vi "Microtrabajo_3.vi"() -> ()   [LabVIEW 2022 SP3]
panel:
  in  "?":enum32{" 1", "2"}(tab)
  in  "?":bool
  out "Fibonacci":string
  in  "Valor límite":dbl
  in  "Stop Button":bool
  in  "DECREMENTAR":bool
  in  "INCREMENTAR":bool
  out "ITERACIONES":string
  out "CUENTA":string
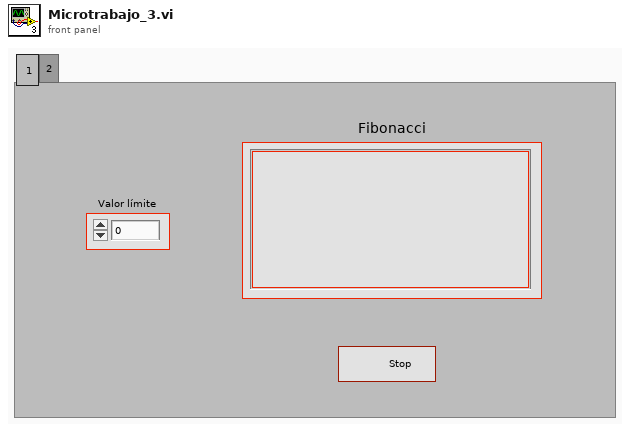
[diagram p1: front panel]
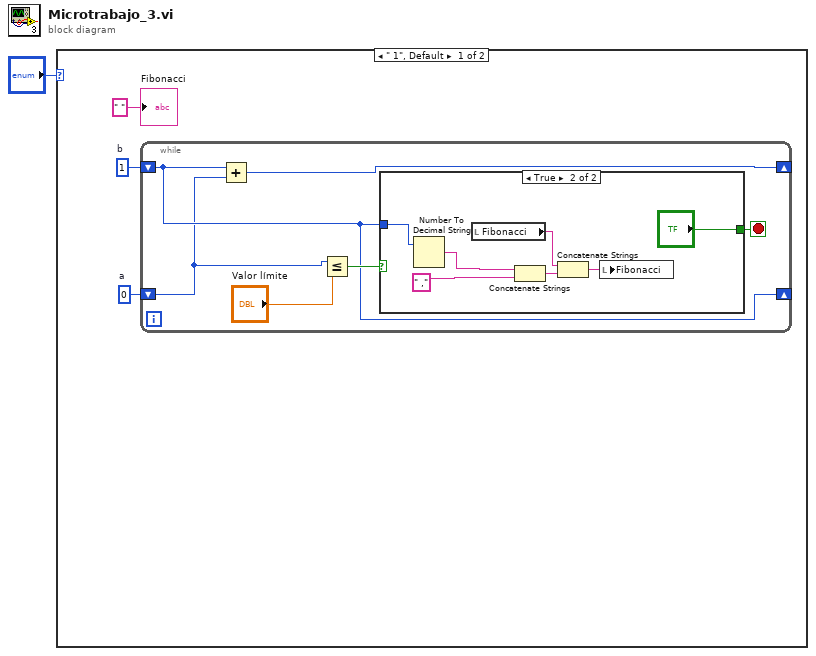
[diagram p0: block diagram]
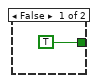
[diagram p2: hidden frame]
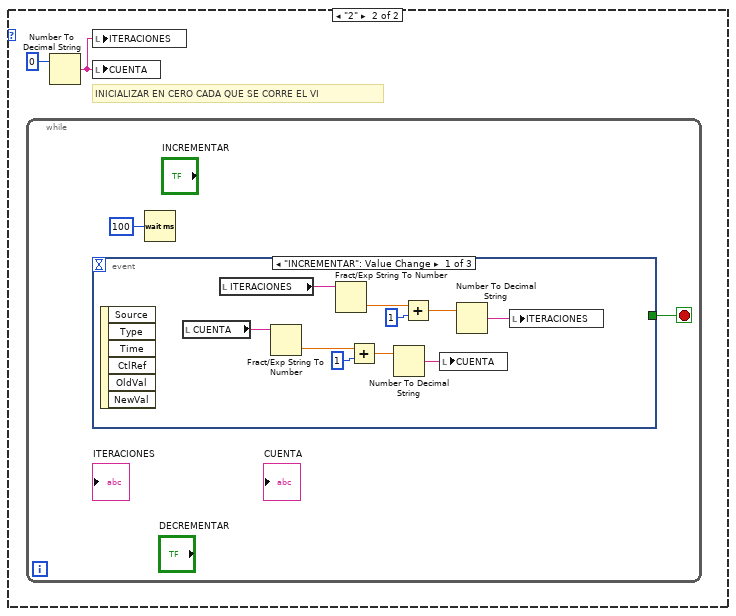
[diagram p3: hidden frame]
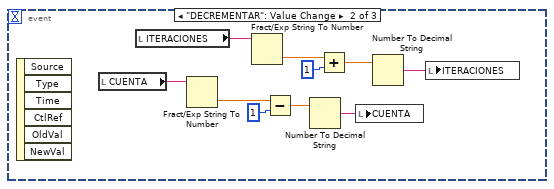
[diagram p4: hidden frame]
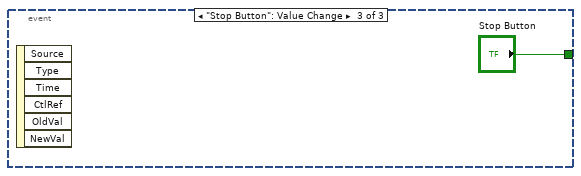
[diagram p5: hidden frame]
diagram:
  n1 = case shown="\" 1\", Default" "?" {
    frame " 1", Default {
      w3 = 0  # a
      w4 = 1  # b
      n2 = while {
        shift-right: [w8] -> _
        shift-left: w4 -> [w7]
        shift-right: [w7] -> _
        shift-left: w3 -> [w5]
        stop <- w6 stop-if-true
        n3 = Add(x=w7, y=w5) -> (x+y=w8:i32)
        n4 = Less Or Equal?(x=w5, y="Valor límite") -> (x <= y?=w9:bool)
        n5 = case shown="True" w9 {
          tunnel: w7 -> [_ w18]
          tunnel: [TRUE "?"] -> w6
          frame False {
          }
          frame True {
            n6 = Number To Decimal String(number=w18) -> (decimal integer string=w12:string)  [unwired: 1 in]
            n7 = local read "Fibonacci"() -> (w15:string)
            n8 = Concatenate Strings(w12, " ,") -> (w14:string)
            n9 = Concatenate Strings(w15, w14) -> (w16:string)
            n10 = local write "Fibonacci"(w16) -> ()
          }
        }
      }
      "Fibonacci" <- " "
    }
    frame "2" {
      # "INICIALIZAR EN CERO CADA QUE SE CORRE EL VI"
      n11 = while {
        stop <- w21 stop-if-true
        n12 = event shown="[0] \"INCREMENTAR\": Value Change" {
          selector: _ -> [_ _ _]
          dyn-events: _ -> [_ _ _]
          timeout: _ -> [_ _ _]
          tunnel: [_ _ "Stop Button"] -> w21
          event "INCREMENTAR": Value Change {
            n13 = event-data() -> ()  [unwired: 1 in, 6 out]
            n14 = local read "CUENTA"() -> (w28:string)
            n15 = local read "ITERACIONES"() -> (w30:string)
            n16 = Fract/Exp String To Number(string=w28) -> (number=w27:dbl)  [unwired: 3 in, 1 out]
            n17 = Fract/Exp String To Number(string=w30) -> (number=w29:dbl)  [unwired: 3 in, 1 out]
            n18 = Add(x=w27, y=1) -> (x+y=w26:dbl)
            n19 = Number To Decimal String(number=w26) -> (decimal integer string=w25:string)  [unwired: 1 in]
            n20 = Add(x=w29, y=1) -> (x+y=w24:dbl)
            n21 = local write "CUENTA"(w25) -> ()
            n22 = Number To Decimal String(number=w24) -> (decimal integer string=w23:string)  [unwired: 1 in]
            n23 = local write "ITERACIONES"(w23) -> ()
          }
          event "DECREMENTAR": Value Change {
            n24 = event-data() -> ()  [unwired: 1 in, 6 out]
            n25 = local read "CUENTA"() -> (w40:string)
            n26 = local read "ITERACIONES"() -> (w42:string)
            n27 = Fract/Exp String To Number(string=w40) -> (number=w35:dbl)  [unwired: 3 in, 1 out]
            n28 = Fract/Exp String To Number(string=w42) -> (number=w41:dbl)  [unwired: 3 in, 1 out]
            n29 = Subtract(x=w35, y=1) -> (x-y=w33:dbl)
            n30 = Number To Decimal String(number=w33) -> (decimal integer string=w39:string)  [unwired: 1 in]
            n31 = Add(x=w41, y=1) -> (x+y=w38:dbl)
            n32 = local write "CUENTA"(w39) -> ()
            n33 = Number To Decimal String(number=w38) -> (decimal integer string=w37:string)  [unwired: 1 in]
            n34 = local write "ITERACIONES"(w37) -> ()
          }
          event "Stop Button": Value Change {
            n35 = event-data() -> ()  [unwired: 1 in, 6 out]
          }
        }
        n36 = Wait (ms)(milliseconds to wait=u32 100) -> ()  [unwired: 1 out]
      }
      n37 = Number To Decimal String(number=0) -> (decimal integer string=w20:string)  [unwired: 1 in]
      n38 = local write "ITERACIONES"(w20) -> ()
      n39 = local write "CUENTA"(w20) -> ()
    }
  }
